vi "Main.vi"(11 "Module Admin":refnum<class "Delacor_lib_QMH_Module Admin.lvclass">) -> ()   [LabVIEW 2019, in "Plantilla.lvlib"]
doc: "This template is based off of the Queued Message Handler design pattern and the Queued Message Handler project template that ships with LabVIEW.\n\nThe main difference is that the queue is private to this module and communication between modules is performed via Broadcast and Request events.\n\nRequest events are wrapped in public API methods and are handled in the Event Handling Loop (EHL) of this VI. Any module can register for Broadcast events sent by this module. The EHL generates messages based on user interface actions.\n\nThe Message Handling Loop (MHL) processes messages generated by the EHL, or by other messages. The messages are string values, so new messages can be added easily to the Message Cases case structure in the MHL. Each message cluster can also provide an optional value for Message Data, which is a variant that can be converted to whatever message-specific data is required.\n_____\nBased on DQMH Dev Tools: Project Template 7.1.0.1503."
uses:
  Plantilla.lvlib
  <vilib>/Delacor/Delacor QMH/Libraries/Module Admin_class/Delacor_lib_QMH_Module Admin.lvclass
  Module Data--cluster.ctl
  <vilib>/Delacor/Delacor QMH/Libraries/Message Queue_class/Delacor_lib_QMH_Message Queue.lvclass/Delacor_lib_QMH_Message Queue.ctl
  Stop Argument--cluster.ctl
  <vilib>/Delacor/Delacor QMH/Libraries/Module Admin_class/Delacor_lib_QMH_Module Admin.lvclass/Delacor_lib_QMH_Module Admin.ctl
  Cambia el color del Panel Argument--cluster.ctl
  <vilib>/Utility/miscctls.llb/LVPointTypeDef.ctl
  <vilib>/Delacor/Delacor QMH/Libraries/Message Queue_class/Delacor_lib_QMH_Enqueue Message (Single).vi
  <vilib>/Delacor/Delacor QMH/Libraries/Module Admin_class/Delacor_lib_QMH_Get External Launch.vi
  <vilib>/Delacor/Delacor QMH/Libraries/Message Queue_class/Delacor_lib_QMH_Message Queue.lvclass
panel:
  out "error out":errorcluster
  out "Status":string
  in  "Simulate MHL Error":bool
  in  "Simulate EHL Error":bool
  # "Other processes communicate with this Module via its Public API (wrappers for its Request Events).\n\nThis Module communicates with other processes via its Broadcast Events.\nAny process that wants to receive these messages can register for this module's Broadcast events."
  # "This template is for the DQMH framework. See the block diagram for more information on how to use this template."
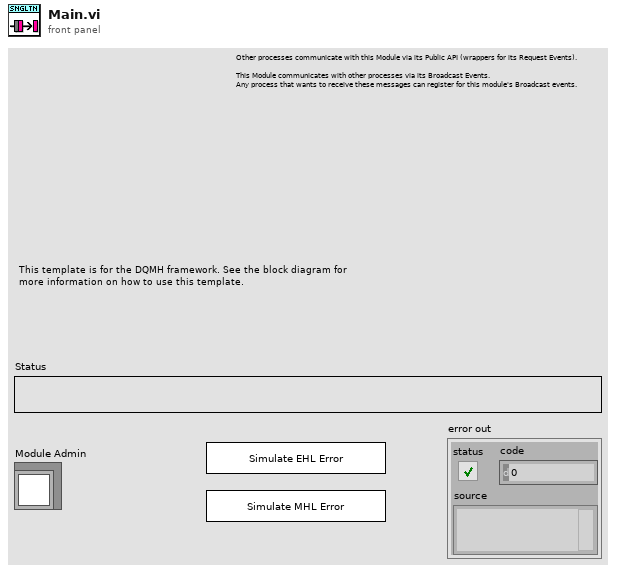
[diagram p1: front panel]
types:
  T1 = typedef "Plantilla.lvlib/Request Events--cluster.ctl" = cluster{"Stop Module":refnum<user-event>, "Show Panel":refnum<user-event>, "Hide Panel":refnum<user-event>, "Get Module Execution Status":refnum<user-event>, "Show Diagram":refnum<user-event>, "Cambia el color del Panel":refnum<user-event>}
  T2 = typedef "Plantilla.lvlib/Module Data--cluster.ctl" = cluster{"Status":string}
  T3 = enum32{"invalid lock state", "Not Locked", "Locked (No Password)", "Password-protected"}
  T4 = typedef "Plantilla.lvlib/Stop Argument--cluster.ctl" = cluster{"Origin":string, "Exit via Stop Module Req?":bool, "Wait for Module to stop?":bool}
  T5 = typedef "Plantilla.lvlib/Cambia el color del Panel Argument--cluster.ctl" = cluster{"Color del Panel":u32}
  T6 = typedef "LVPointTypeDef.ctl" = cluster{"Horizontal":i16, "Vertical":i16}
  T7 = enum32{"Invalid", "Standard", "Closed", "Hidden", "Minimized", "Maximized"}
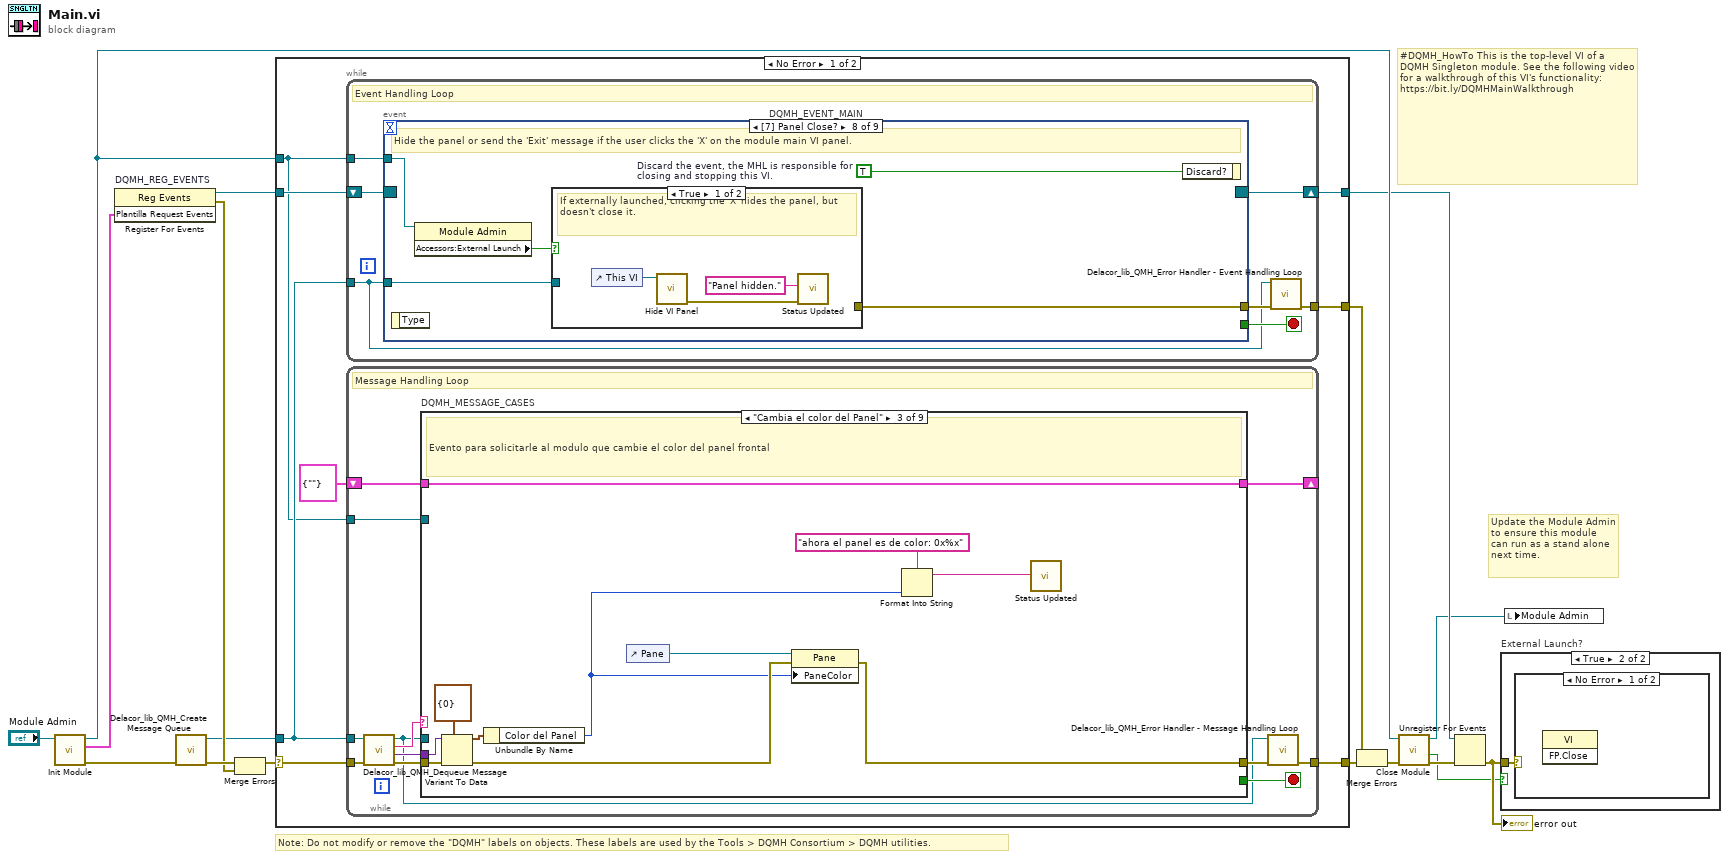
[diagram p0: block diagram]
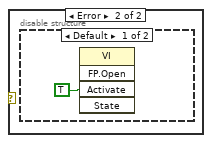
[diagram p3: hidden frame]
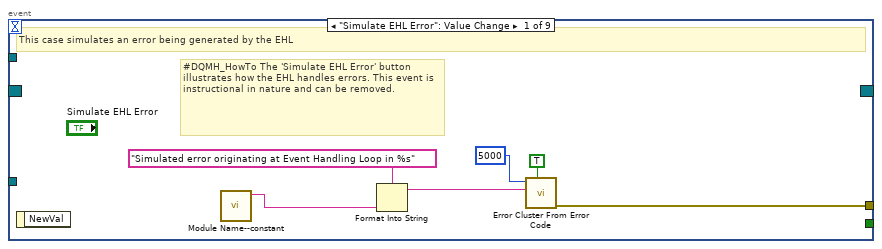
[diagram p5: hidden frame]
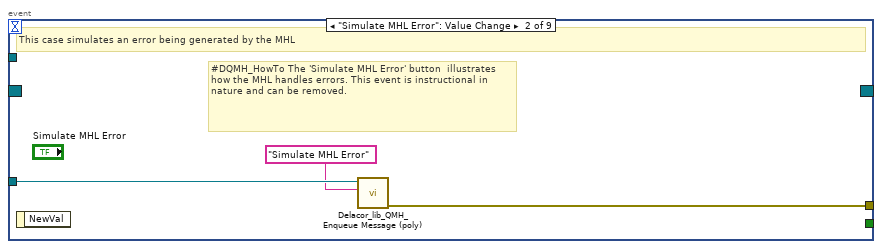
[diagram p6: hidden frame]
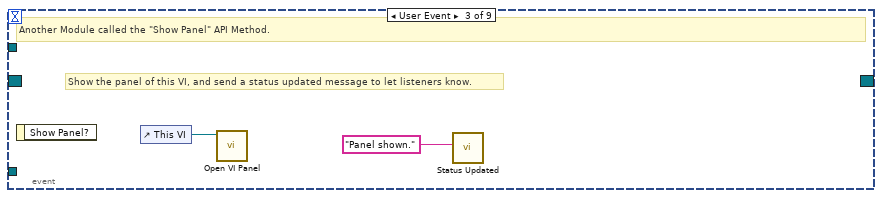
[diagram p7: hidden frame]
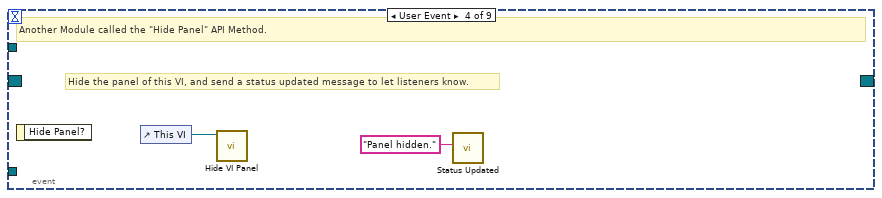
[diagram p8: hidden frame]
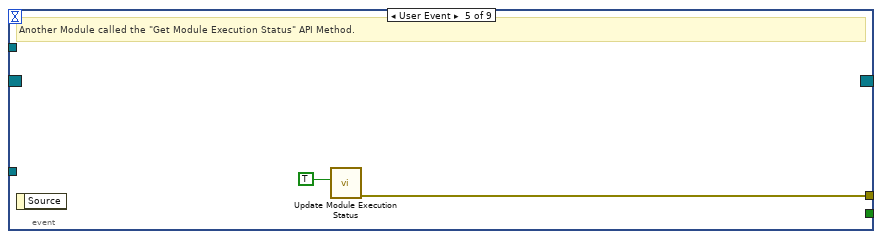
[diagram p9: hidden frame]
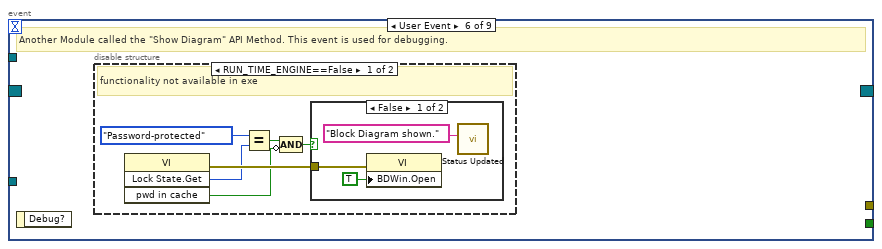
[diagram p10: hidden frame]
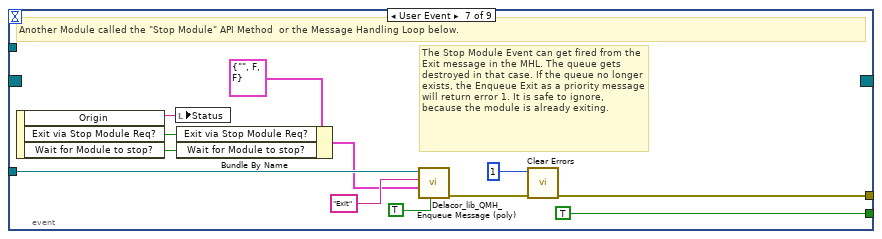
[diagram p13: hidden frame]
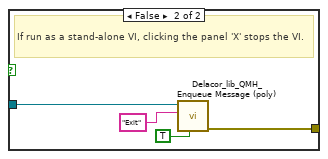
[diagram p14: hidden frame]
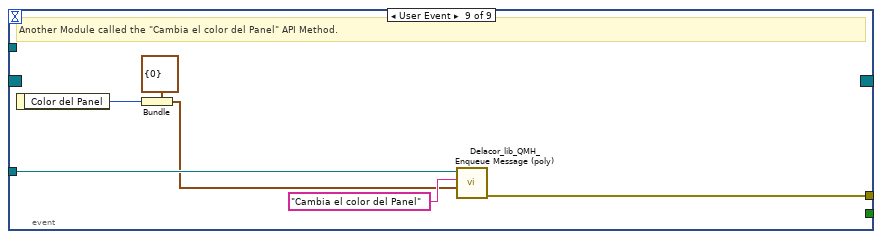
[diagram p15: hidden frame]
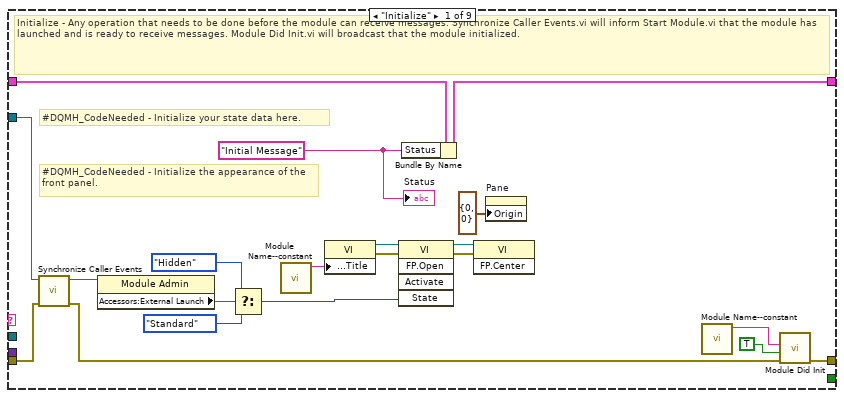
[diagram p16: hidden frame]
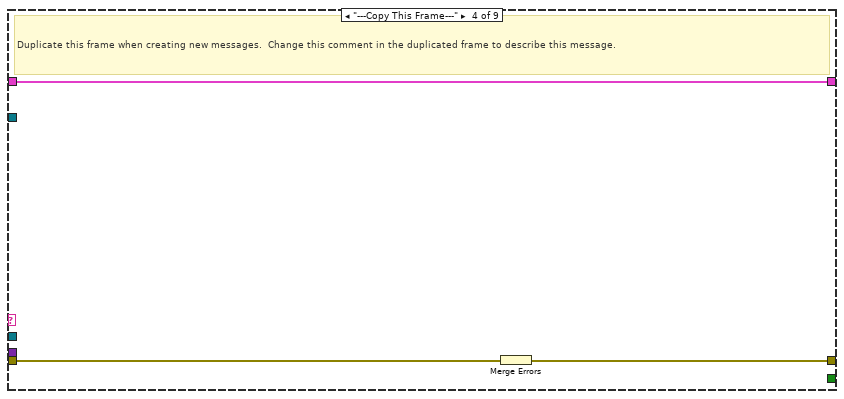
[diagram p18: hidden frame]
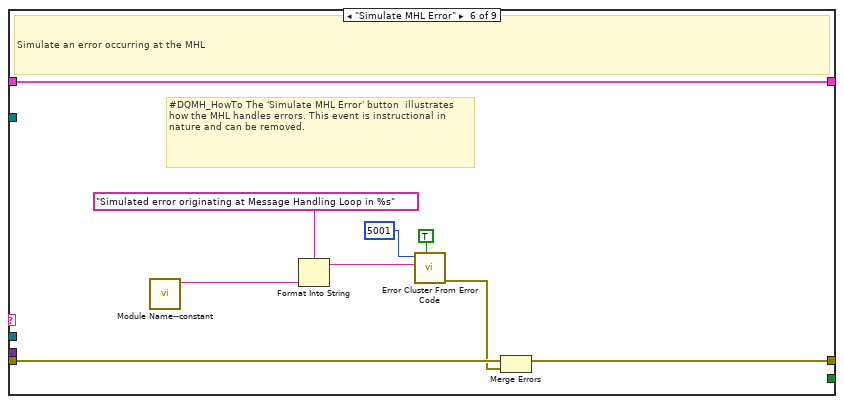
[diagram p20: hidden frame]
diagram:
  # "#DQMH_HowTo This is the top-level VI of a DQMH Singleton module. See the following video for a walkthrough of this VI's functionality: https://bit.ly/DQMHMainWalkthrough"
  # "Note: Do not modify or remove the \"DQMH\" labels on objects. These labels are used by the Tools > DQMH Consortium > DQMH utilities."
  # "Update the Module Admin to ensure this module can run as a stand alone next time."
  n1 = call "Init Module.vi"("Singleton Module Admin in"="Module Admin") -> ("error out"=w16:errorcluster, "Plantilla Request Events"=w5:T1, "Singleton Module Admin out"=w8:refnum<class "Delacor_lib_QMH_Module Admin.lvclass">)  [unwired: 8 in]
  n2 = register-events "DQMH_REG_EVENTS"(w5) -> (reference out=w6:refnum<event-registration>, error out=w9:errorcluster)  [unwired: 2 in]
  n3 = call <vilib>:"Delacor_lib_QMH_Create Message Queue.vi"("error in"=w16) -> ("error out"=w11:errorcluster, "Message Queue"=w4:refnum<class "Delacor_lib_QMH_Message Queue.lvclass">)  [unwired: 9 in]
  n4 = Merge Errors(w11, w9) -> (w10:errorcluster)
  n5 = case shown="No Error" w10 {
    selector: w10 -> [w23 w195]
    tunnel: [w25 w194] -> w17
    tunnel: [w22 w193] -> w7
    tunnel: w6 -> [w20 w193]
    tunnel: w4 -> [w19 w188]
    tunnel: [w24 _] -> w14
    tunnel: w8 -> [w18 w189]
    frame No Error {
      n6 = while {
        tunnel: w19 -> [w26]
        shift-right: [w29] -> w22
        shift-left: w20 -> [w30]
        tunnel: [w31] -> w24
        tunnel: w18 -> [w27]
        stop <- w28 stop-if-true
        # "Event Handling Loop"
        n7 = event "DQMH_EVENT_MAIN" shown="[7] Panel Close?" {
          selector: w30 -> [_ _ _ _ _ _ _ _ _]
          dyn-events: [_ _ _ _ _ _ _ _ _] -> w29
          timeout: _ -> [_ _ _ _ _ _ _ _ _]
          tunnel: [_ _ _ _ _ _ TRUE ("Discard?") _ _] -> w28
          tunnel: w26 -> [_ w40 _ _ _ _ w64 w71 w86]
          tunnel: [w38 w41 _ _ w47 _ w67 w73 w81] -> w32
          tunnel: w27 -> [_ _ _ _ _ _ _ w70 _]
          event "Simulate EHL Error": Value Change {
            # "#DQMH_HowTo The 'Simulate EHL Error' button  illustrates how the EHL handles errors. This event is instructional in nature and can be removed."
            # "This case simulates an error being generated by the EHL"
            n8 = event-data() -> ()  [unwired: 1 in, 1 out]
            n9 = call "Module Name--constant.vi"() -> ("Module Name"=w35:string)  [unwired: 11 in]
            n10 = Format Into String(format string="Simulated error originating at Event Handling Loop in %s", w35) -> (resulting string=w36:string)  [unwired: 2 in, 1 out]
            n11 = call <vilib>:"Error Cluster From Error Code.vi"("show call chain? (False)"=TRUE, "error message (\"\")"=w36, "error code (0)"=5000) -> ("error out"=w38:errorcluster)  [unwired: 6 in]
          }
          event "Simulate MHL Error": Value Change {
            # "#DQMH_HowTo The 'Simulate MHL Error' button  illustrates how the MHL handles errors. This event is instructional in nature and can be removed."
            # "This case simulates an error being generated by the MHL"
            n12 = event-data() -> ()  [unwired: 1 in, 1 out]
            n13 = call-poly <vilib>:"Delacor_lib_QMH_Enqueue Message (poly).vi"("Message"="Simulate MHL Error", "Message Queue in"=w40) -> ("error out"=w41:errorcluster)  [unwired: 8 in, 1 out]
          }
          event User Event {
            # "Show the panel of this VI, and send a status updated message to let listeners know."
            # "Another Module called the \"Show Panel\" API Method."
            n14 = event-data() -> ()  [unwired: 1 in, 1 out]
            n15 = control-ref of="This VI"() -> (w43:refnum<vi>)
            n16 = call "Open VI Panel.vi"("VI"=w43) -> ()  [unwired: 10 in, 1 out]
            n17 = call "Status Updated.vi"("Status"="Panel shown." ("format string")) -> ()  [unwired: 10 in, 1 out]
          }
          event User Event {
            # "Hide the panel of this VI, and send a status updated message to let listeners know."
            # "Another Module called the \"Hide Panel\" API Method."
            n18 = event-data() -> ()  [unwired: 1 in, 1 out]
            n19 = control-ref of="This VI"() -> (w45:refnum<vi>)
            n20 = call "Hide VI Panel.vi"("VI"=w45) -> ()  [unwired: 10 in, 1 out]
            n21 = call "Status Updated.vi"("Status"="Panel hidden." ("format string")) -> ()  [unwired: 10 in, 1 out]
          }
          event User Event {
            # "Another Module called the \"Get Module Execution Status\" API Method."
            n22 = event-data() -> ()  [unwired: 1 in, 1 out]
            n23 = call "Update Module Execution Status.vi"("Running?"=TRUE) -> ("error out"=w47:errorcluster)  [unwired: 10 in]
          }
          event User Event {
            # "Another Module called the \"Show Diagram\" API Method. This event is used for debugging."
            n24 = event-data() -> ()  [unwired: 1 in, 1 out]
            n25 = disable-structure shown="RUN_TIME_ENGINE==False" {
              frame condition #0 (active) {
                # "functionality not available in exe"
                n26 = invoke on="Invoke Node" class="VI" method="Lock State.Get"() -> (error out=w53:errorcluster, "Get Lock State"=w52:T3, "pwd in cache"=w49:bool)  [unwired: 4 in, 1 out]
                n27 = Equal?(x=T3."Password-protected", y=w52) -> (x = y?=w50:bool)
                n28 = Compound Arithmetic op=AND(w50, invert w49) -> (w48:bool)
                n29 = case shown="False" w48 {
                  tunnel: w53 -> [w56 _]
                  frame False {
                    n30 = property on="Property Node" class="VI"(error in=w56, "BDWin.Open"=TRUE ("Block Diagram Window:Open")) -> ()  [unwired: 1 in, 2 out]
                    n31 = call "Status Updated.vi"("Status"="Block Diagram shown." ("format string")) -> ()  [unwired: 10 in, 1 out]
                  }
                  frame True {
                    # "Password-protected VI, and the password is not in the cache. Do not show the diagram."
                  }
                }
              }
              frame condition #1 {
              }
            }
          }
          event User Event {
            # "The Stop Module Event can get fired from the Exit message in the MHL. The queue gets destroyed in that case. If the queue no longer exists, the Enqueue Exit as a priority message will return error 1. It is safe to ignore, because the module is already exiting."
            # "Another Module called the \"Stop Module\" API Method  or the Message Handling Loop below."
            n32 = event-data() -> ("Origin"=w63:string, "Exit via Stop Module Req?"=w59:bool, "Wait for Module to stop?"=w58:bool)  [unwired: 1 in]
            n33 = local write "Status"(w63) -> ()
            n34 = Bundle By Name(cluster=T4 {"Origin"="", "Exit via Stop Module Req?"=FALSE, "Wait for Module to stop?"=FALSE} ("Stop Argument"), "Exit via Stop Module Req?"=w59, "Wait for Module to stop?"=w58) -> (w57:T4)
            n35 = call-poly <vilib>:"Delacor_lib_QMH_Enqueue Message (poly).vi"("Priority Message? (F)"=TRUE, "Message Data"=w57, "Message"="Exit", "Message Queue in"=w64) -> ("error out"=w68:errorcluster)  [unwired: 6 in, 1 out]
            n36 = call <vilib>:"Clear Errors.vi"("error in (no error)"=w68, "specific error code to clear (0: all)"=1) -> ("error out"=w67:errorcluster)  [unwired: 4 in, 1 out]
          }
          event Panel Close? {
            w72 = TRUE  # Discard the event, the MHL is responsible for closing and stopping this VI.
            # "Hide the panel or send the 'Exit' message if the user clicks the 'X' on the module main VI panel."
            n37 = event-data() -> ()  [unwired: 1 in, 1 out]
            n38 = property on="Property Node" class="Module Admin"(reference=w70) -> ("Accessors:External Launch"=w69:bool)  [unwired: 1 in, 2 out]
            n39 = case shown="True" w69 {
              tunnel: w71 -> [_ w79]
              tunnel: [_ w80] -> w73
              frame True {
                # "If externally launched, clicking the 'X' hides the panel, but doesn't close it."
                n40 = control-ref of="This VI"() -> (w76:refnum<vi>)
                n41 = call "Hide VI Panel.vi"("VI"=w76) -> ("error out"=w74:errorcluster)  [unwired: 10 in]
                n42 = call "Status Updated.vi"("error in"=w74, "Status"="Panel hidden." ("format string")) -> ()  [unwired: 9 in, 1 out]
              }
              frame False {
                # "If run as a stand-alone VI, clicking the panel 'X' stops the VI."
                n43 = call-poly <vilib>:"Delacor_lib_QMH_Enqueue Message (poly).vi"("Priority Message? (F)"=TRUE, "Message"="Exit", "Message Queue in"=w79) -> ("error out"=w80:errorcluster)  [unwired: 7 in, 1 out]
              }
            }
            n44 = event-data ("Event Filter Node")("Discard?"=w72) -> ()  [unwired: 1 in, 1 out]
          }
          event User Event {
            # "Another Module called the \"Cambia el color del Panel\" API Method."
            n45 = event-data() -> ("Color del Panel"=w82:u32)  [unwired: 1 in]
            n46 = Bundle(cluster=T5 {"Color del Panel"=0} ("Cambia el color del Panel Argument"), "Color del Panel"=w82) -> (w83:T5)
            n47 = call-poly <vilib>:"Delacor_lib_QMH_Enqueue Message (poly).vi"("Message Data"=w83, "Message"="Cambia el color del Panel", "Message Queue in"=w86) -> ("error out"=w81:errorcluster)  [unwired: 7 in, 1 out]
          }
        }
        n48 = call-dynamic "Delacor_lib_QMH_Error Handler - Event Handling Loop.vi"("error in"=w32, "Message Queue in"=w26) -> ("dup error in"=w31:errorcluster)  [unwired: 8 in, 1 out]
      }
      n49 = while {
        tunnel: w19 -> [w87]
        shift-right: [w95] -> _
        shift-left: T2 {"Status"=""} ("Data Cluster") -> [w96]
        tunnel: w23 -> [w98]
        tunnel: [w90] -> w25
        tunnel: w18 -> [w91]
        stop <- w94 stop-if-true
        # "Message Handling Loop"
        n50 = call-dynamic "Delacor_lib_QMH_Dequeue Message.vi"("error in"=w98, "Message Queue in"=w87) -> ("error out"=w97:errorcluster, "Message Data"=w92:variant, "Message"=w93:string, "Message Queue out"=w88:refnum<class "Delacor_lib_QMH_Message Queue.lvclass">)  [unwired: 6 in]
        n51 = case "DQMH_MESSAGE_CASES" shown="\"Cambia el color del Panel\"" w93 {
          selector: w93 -> [_ _ _ _ _ _ _ _ w183]
          tunnel: w88 -> [_ _ _ _ _ _ w149 w171 _]
          tunnel: w97 -> [w116 w120 w131 w134 w136 w145 w156 w177 w186]
          tunnel: [w114 w120 w124 w133 w136 w144 w152 w172 w187] -> w89
          tunnel: w96 -> [w105 w119 w130 w132 w135 w142 w151 w170 w184]
          tunnel: [w104 w119 w130 w132 w135 w142 w151 w170 w184] -> w95
          tunnel: [_ _ _ _ _ _ _ w169 _] -> w94
          tunnel: w92 -> [_ _ w129 _ _ _ w150 w168 _]
          tunnel: w91 -> [w106 _ _ _ _ _ w148 w163 _]
          frame "Initialize" {
            w100 = "Initial Message" ("Initial Message")
            # "#DQMH_CodeNeeded - Initialize the appearance of the front panel."
            # "#DQMH_CodeNeeded - Initialize your state data here."
            # "Initialize - Any operation that needs to be done before the module can receive messages. Synchronize Caller Events.vi will inform Start Module.vi that the module has launched and is ready to receive messages. Module Did Init.vi will broadcast that the module initialized."
            n52 = call "Synchronize Caller Events.vi"("error in"=w116, "Singleton Module Admin in"=w106) -> ("error out"=w115:errorcluster, "Singleton Module Admin out"=w101:refnum<class "Delacor_lib_QMH_Module Admin.lvclass">)  [unwired: 8 in]
            n53 = property on="Property Node" class="Module Admin"(reference=w101) -> ("Accessors:External Launch"=w110:bool)  [unwired: 1 in, 2 out]
            n54 = Select(t=T7."Hidden" ("State"), s=w110, f=T7."Standard" ("State")) -> (s? t:f=w107:T7)
            n55 = call "Module Name--constant.vi"() -> ("Module Name"=w113:string)  [unwired: 11 in]
            n56 = property on="Property Node" class="VI"("Front Panel.Title"=w113) -> (reference out=w112:refnum<vi>, error out=w118:errorcluster)  [unwired: 2 in]
            n57 = invoke on="Invoke Node" class="VI" method="FP.Open"(reference=w112, error in=w118, "State"=w107) -> (reference out=w111:refnum<vi>, error out=w117:errorcluster)  [unwired: 2 in, 3 out]
            n58 = Bundle By Name(cluster=w105, "Status"=w100) -> (w104:T2)
            n59 = invoke on="Invoke Node" class="VI" method="FP.Center"(reference=w111, error in=w117) -> ()  [unwired: 1 in, 3 out]
            n60 = property on="Pane" class="Pane"("Origin"=T6 {"Horizontal"=0, "Vertical"=0}) -> ()  [unwired: 2 in, 2 out]
            n61 = call "Module Name--constant.vi"() -> ("Module Name"=w102:string)  [unwired: 11 in]
            n62 = call "Module Did Init.vi"("error in"=w115, "Initialized?"=TRUE, "Origin"=w102) -> ("error out"=w114:errorcluster)  [unwired: 8 in]
            "Status" <- w100
          }
          frame "---Module Specific---" {
            # "Separator -- The following cases handle messages specific to this Module."
          }
          frame "Cambia el color del Panel" {
            # "Evento para solicitarle al modulo que cambie el color del panel frontal"
            n63 = Variant To Data(error in=w131, type=T5 {"Color del Panel"=0} ("Cambia el color del Panel Argument"), Variant=w129) -> (data=w127:T5, error out=w125:errorcluster)
            n64 = Unbundle By Name(w127) -> ("Color del Panel"=w123:u32)
            n65 = control-ref of="Pane"() -> (w126:refnum<vi>)
            n66 = property class="Pane"(reference=w126, error in=w125, "PaneColor"=w123) -> (error out=w124:errorcluster)  [unwired: 1 out]
            n67 = Format Into String(format string="ahora el panel es de color: 0x%x", w123) -> (resulting string=w122:string)  [unwired: 2 in, 1 out]
            n68 = call "Status Updated.vi"("Status"=w122) -> ()  [unwired: 10 in, 1 out]
          }
          frame "---Copy This Frame---" {
            # "Duplicate this frame when creating new messages.  Change this comment in the duplicated frame to describe this message."
            n69 = Merge Errors(w134) -> (w133:errorcluster)
          }
          frame "---Exit and Error Handling---" {
            # "Separator - The following cases handle errors and exit messages."
          }
          frame "Simulate MHL Error" {
            # "#DQMH_HowTo The 'Simulate MHL Error' button  illustrates how the MHL handles errors. This event is instructional in nature and can be removed."
            # "Simulate an error occurring at the MHL"
            n70 = call "Module Name--constant.vi"() -> ("Module Name"=w138:string)  [unwired: 11 in]
            n71 = Format Into String(format string="Simulated error originating at Message Handling Loop in %s", w138) -> (resulting string=w139:string)  [unwired: 2 in, 1 out]
            n72 = call <vilib>:"Error Cluster From Error Code.vi"("show call chain? (False)"=TRUE, "error message (\"\")"=w139, "error code (0)"=5001) -> ("error out"=w143:errorcluster)  [unwired: 6 in]
            n73 = Merge Errors(w145, w143) -> (w144:errorcluster)
          }
          frame "Error" {
            # "#DQMH_CodeRecommended - If the module is running in standalone mode (External Launch = FALSE), this code will pop up an error dialog and call the 'Exit' message if an error occurs. Add more fine-grained error management here."
            # "Error - Check the error message data and respond accordingly. This message is sent by the \"Error Handler\" VIs at the end of each loop in this application."
            n74 = property on="Property Node" class="Module Admin"(reference=w148) -> ("Accessors:External Launch"=w147:bool)  [unwired: 1 in, 2 out]
            n75 = Variant To Data(error in=w156, type=errorcluster {"status"=FALSE, "code"=0, "source"=""} ("error constant"), Variant=w150) -> (data=w146:errorcluster, error out=w154:errorcluster)
            n76 = local write "error out"(w146) -> ()
            n77 = call "Error Reported.vi"("Error"=w146) -> ()  [unwired: 10 in, 1 out]
            n78 = case shown="False" w147 {
              tunnel: [w161 _] -> w153
              tunnel: w149 -> [w159 _]
              tunnel: w146 -> [w160 _]
              frame False {
                n79 = disable-structure shown="Default" {
                  disable-tunnel: w160 -> [w162 _]
                  frame condition #0 (active) {
                    # "If the module is running standalone, then pop up an error dialog and call the \"Exit\" message."
                    n80 = call <vilib>:"Simple Error Handler.vi"("error in (no error)"=w162) -> ()  [unwired: 4 in, 5 out]
                  }
                  frame condition #1 {
                    # "To prevent the Simple Error Handler VI from being loaded (e.g. when deploying to a Real-Time target), add the Conditional Disable Symbol \"DQMH_Disable_SEH\" to your project and set it to TRUE."
                  }
                }
                n81 = call-poly <vilib>:"Delacor_lib_QMH_Enqueue Message (poly).vi"("Priority Message? (F)"=TRUE, "Message"="Exit", "Message Queue in"=w159) -> ("error out"=w161:errorcluster)  [unwired: 7 in, 1 out]
              }
              frame True {
                # "If the module was launched externally, calling the Error Reported broadcast VI is the only action performed by the \"Error\" message. The module's caller can then process the error appropriately."
              }
            }
            n82 = Merge Errors(w154, w153) -> (w152:errorcluster)
          }
          frame "Exit" {
            w167 = 91  # 91: not all Exit messages will have an argument
            w169 = TRUE  # Stop the VI
            # "Release the message queue reference"
            # "#DQMH_CodeNeeded - Add any required cleanup code here."
            # "Exit - Exit the application."
            n83 = Variant To Data(error in=w177, type=T4 {"Origin"="", "Exit via Stop Module Req?"=FALSE, "Wait for Module to stop?"=FALSE} ("Stop Argument"), Variant=w168) -> (data=w165:T4, error out=w174:errorcluster)
            n84 = call <vilib>:"Clear Errors.vi"("error in (no error)"=w174, "specific error code to clear (0: all)"=w167) -> ("error out"=w176:errorcluster)  [unwired: 4 in, 1 out]
            n85 = control-ref of="This VI"() -> (w164:refnum<vi>)
            n86 = call-dynamic "Delacor_lib_QMH_Release Message Queue.vi"("error in"=w176, "Message Queue"=w171) -> ("error out"=w175:errorcluster)  [unwired: 9 in]
            n87 = call "Handle Exit.vi"("Stop Argument"=w165, "Admin in"=w163, "VI reference"=w164) -> ("error out"=w173:errorcluster)  [unwired: 7 in, 1 out]
            n88 = Merge Errors(w175, w173) -> (w172:errorcluster)
            n89 = call "Error Reported.vi"("Error"=w172) -> ()  [unwired: 10 in, 1 out]
          }
          frame Default {
            # "'Default' case only runs if there is a message that isn't defined in any of the other cases.  Output a programming error."
            n90 = call "Module Name--constant.vi"() -> ("Module Name"=w182:string)  [unwired: 11 in]
            n91 = Format Into String(format string="The invalid message string \"%s\" was received in the Message Handling Loop for module \"%s\".", w183, w182) -> (resulting string=w178:string)  [unwired: 2 in, 1 out]
            n92 = call <vilib>:"Error Cluster From Error Code.vi"("show call chain? (False)"=TRUE, "error message (\"\")"=w178, "error code (0)"=1) -> ("error out"=w185:errorcluster)  [unwired: 6 in]
            n93 = Merge Errors(w186, w185) -> (w187:errorcluster)
          }
        }
        n94 = call-dynamic "Delacor_lib_QMH_Error Handler - Message Handling Loop.vi"("error in"=w89, "Message Queue in"=w88) -> ("dup error in"=w90:errorcluster)  [unwired: 8 in, 1 out]
      }
    }
    frame Error {
      # "Synchronize Caller Events.vi will inform Start Module.vi that the module has launched and will let the code calling Start Module.vi register for broadcasts and would permit the caller receive the broadcast that an error occurred at launch time."
      n95 = call-dynamic "Delacor_lib_QMH_Release Message Queue.vi"("error in"=w195, "Message Queue"=w188) -> ("error out"=w194:errorcluster)  [unwired: 9 in]
      n96 = call "Synchronize Caller Events.vi"("Singleton Module Admin in"=w189) -> ("error out"=w196:errorcluster)  [unwired: 9 in, 1 out]
      n97 = call "Module Name--constant.vi"() -> ("Module Name"=w192:string)  [unwired: 11 in]
      n98 = Format Into String(format string="An error occurred during initialization. %s is no longer running.", w192) -> (resulting string=w190:string)  [unwired: 2 in, 1 out]
      n99 = Merge Errors(w194, w196) -> (w197:errorcluster)
      n100 = call "Error Reported.vi"("Additional Information"=w190, "Error"=w197) -> ()  [unwired: 9 in, 1 out]
    }
  }
  n101 = Merge Errors(w14, w17) -> (w13:errorcluster)
  n102 = call "Close Module.vi"("error in"=w13, "Module Admin in"=w8) -> ("error out"=w15:errorcluster, "External Launch"=w1:bool, "Module Admin out"=w2:refnum<class "Delacor_lib_QMH_Module Admin.lvclass">)  [unwired: 7 in]
  n103 = Unregister For Events(event registration refnum=w7, error in=w15) -> (error out=w12:errorcluster)
  "error out" <- w12
  n104 = case "External Launch?" shown="True" w1 {
    tunnel: w12 -> [_ w198]
    frame False {
    }
    frame True {
      n105 = case shown="No Error" w198 {
        frame No Error {
          n106 = invoke on="Invoke Node" class="VI" method="FP.Close"() -> ()  [unwired: 3 in, 3 out]
        }
        frame Error {
          n107 = disable-structure shown="Default" {
            frame condition #0 (active) {
              n108 = invoke class="VI" method="FP.Open"("Activate"=TRUE ("Activate?")) -> ()  [unwired: 4 in, 5 out]
            }
            frame condition #1 {
              # "Don't show panel on error if running inside a built EXE."
            }
          }
        }
      }
    }
  }
  n109 = local write "Module Admin"(w2) -> ()
